vi "校准任务设置.vi"(9 "精度":dbl=4.0, 10 "模型":enum32{"线性", "多项式"}(ring), 11 "用户事件":refnum<user-event>) -> ()   [LabVIEW 2016, in "斯坦道氨氮.lvlib"]
panel:
  in  "校准任务存档":T1[](array[typedef])
  out "字符串":string
  out "校准运行状态":bool
  in  "校准任务":T1[](array[typedef])
  in  "停止":bool
  in  "设置":bool
  in  "执行":bool
  in  "删除":bool
  in  "清空":bool
  in  "任务列表":i32(listbox)
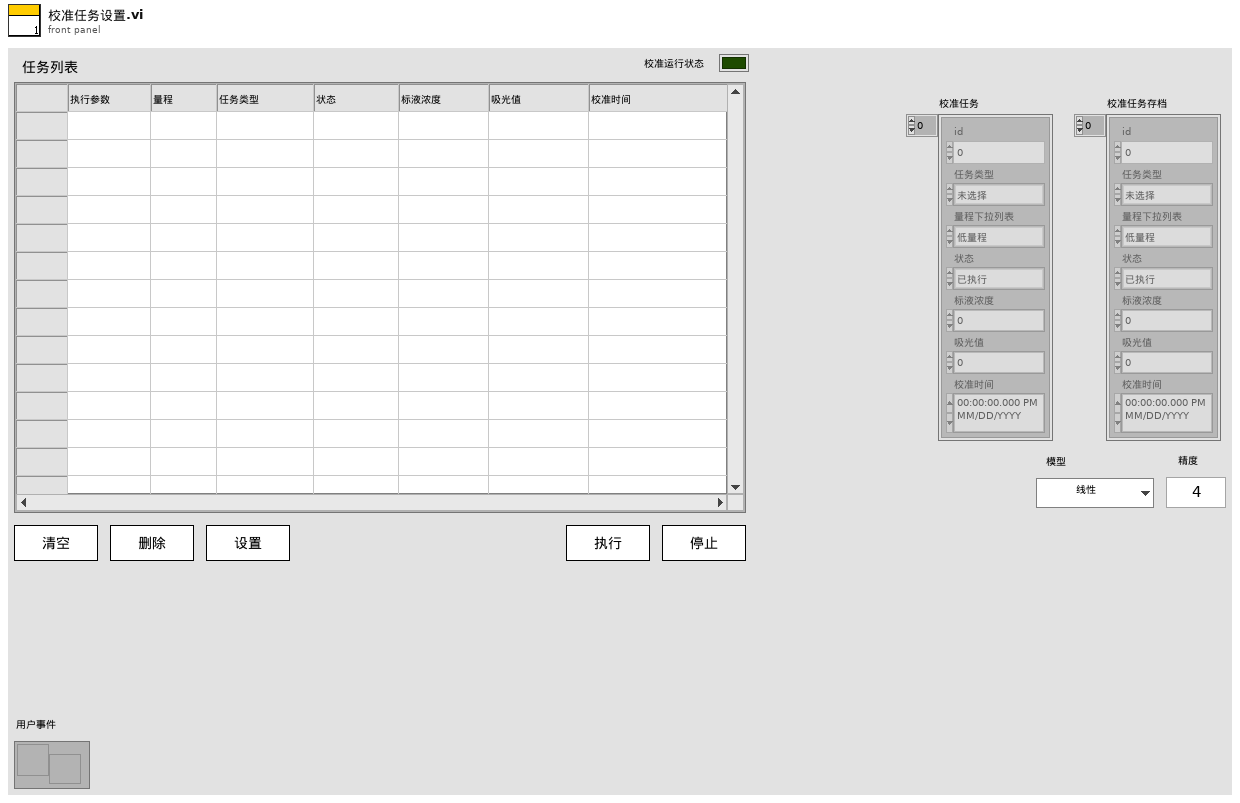
[diagram p1: front panel]
types:
  T1 = typedef "斯坦道氨氮.lvlib/校准任务.ctl" = cluster{"id":u16, "任务类型":enum16{"未选择", "空白校准", "标样校准", "标样核查", "零点核查", "跨度核查"}, "量程下拉列表":enum16{"低量程", "高量程"}, "状态":enum16{"已执行", "待执行", "执行中", "停止"}, "标液浓度":dbl, "吸光值":dbl, "校准时间":timestamp}
  T2 = cluster{"校准类型":string, "校准数据":cluster{"时间":timestamp, "标液值":dbl, "检测值":dbl, "吸光值":dbl}}
  T3 = enum8{"Enabled", "Disabled", "Disabled and Grayed Out"}
  T4 = typedef "LVPoint32TypeDef.ctl" = cluster{"Horizontal":i32, "Vertical":i32}
  T5 = typedef "LVRowAndColumnTypeDef.ctl" = cluster{"Row":i32, "Column":i32}
  T6 = enum16{"未选择", "空白校准", "标样校准", "标样核查", "零点核查", "跨度核查"}
  T7 = cluster{"id":u16, "任务类型":enum16{"未选择", "空白校准", "标样校准", "标样核查", "零点核查", "跨度核查"}, "量程下拉列表":enum16{"低量程", "高量程"}, "状态":enum16{"已执行", "待执行", "执行中", "停止"}, "标液浓度":dbl, "吸光值":dbl, "校准时间":timestamp}
  T8 = enum32{"Bad", "Idle", "Run top level", "Running"}
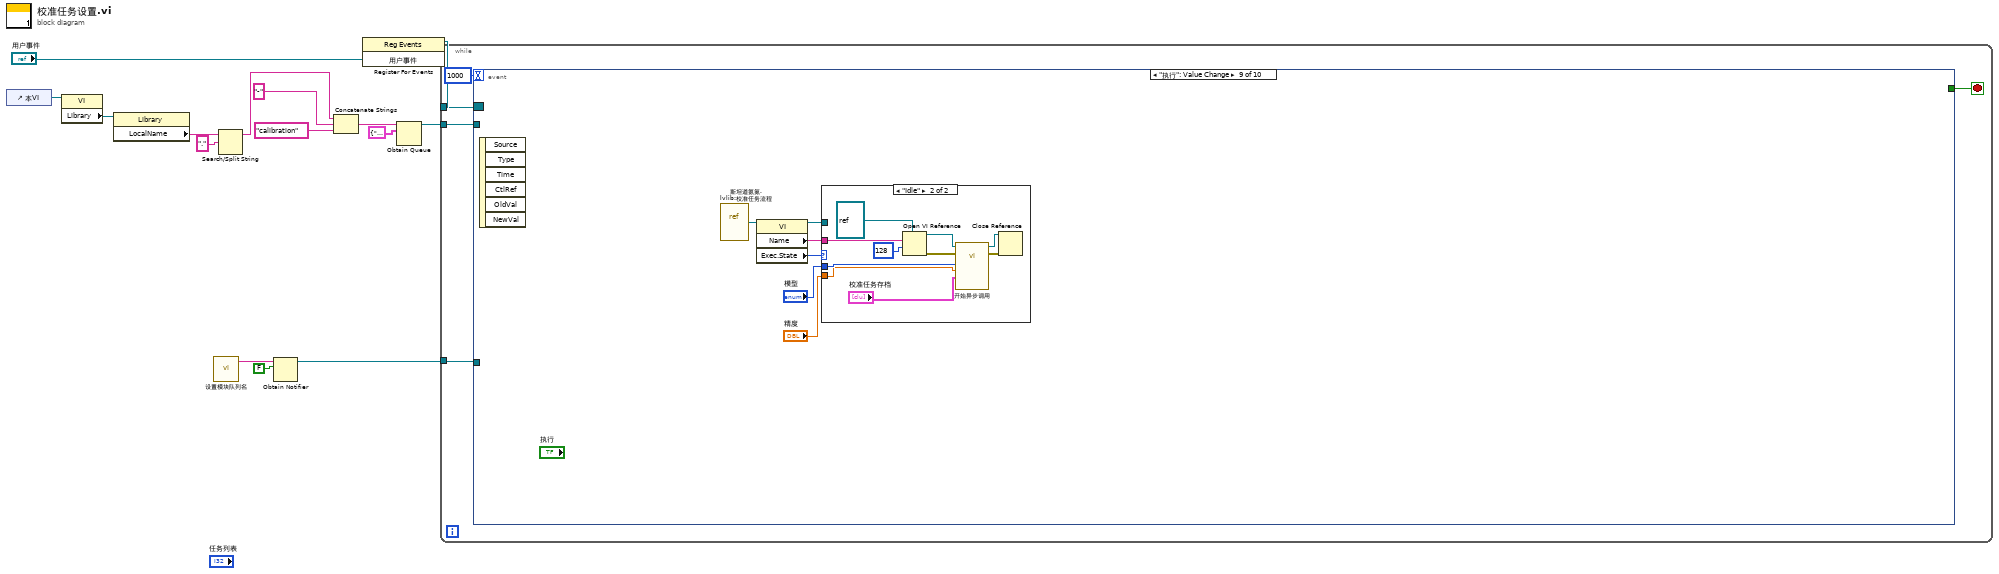
[diagram p0: block diagram]
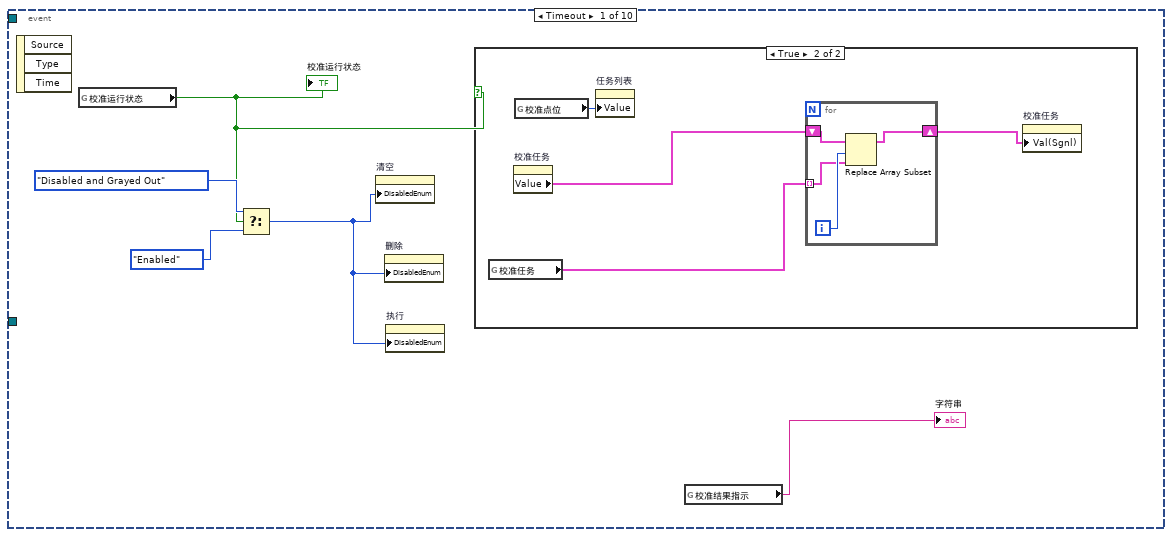
[diagram p2: hidden frame]
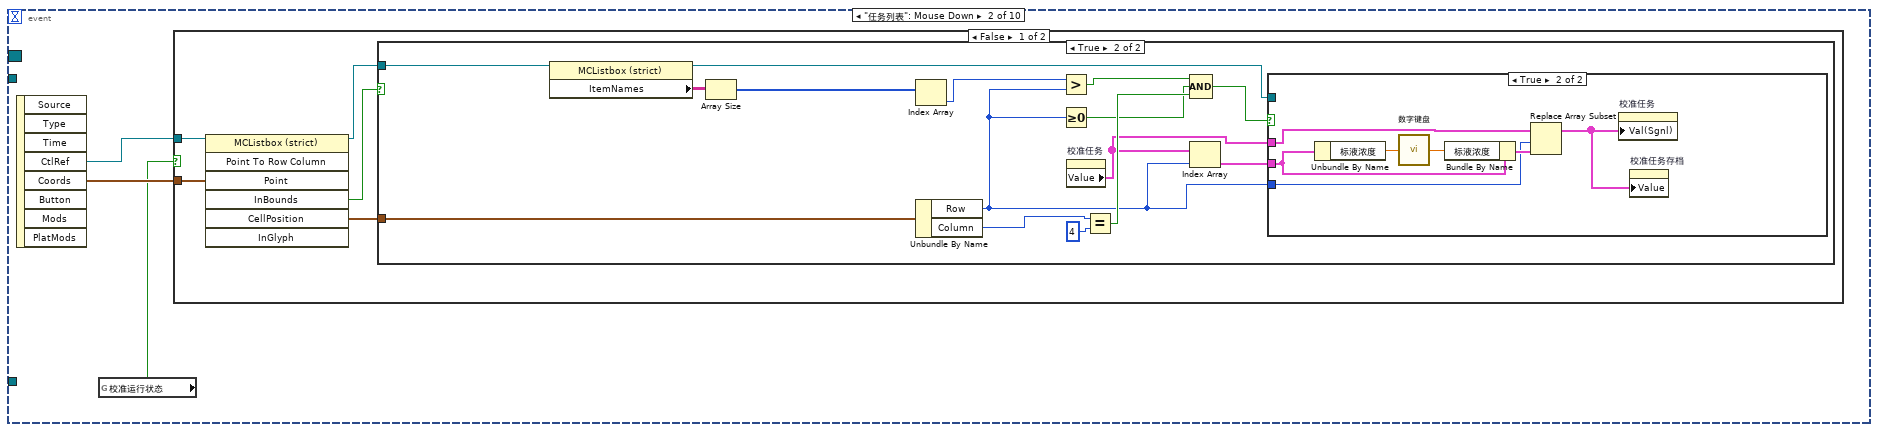
[diagram p4: hidden frame]
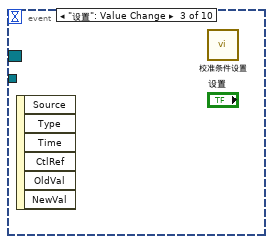
[diagram p8: hidden frame]
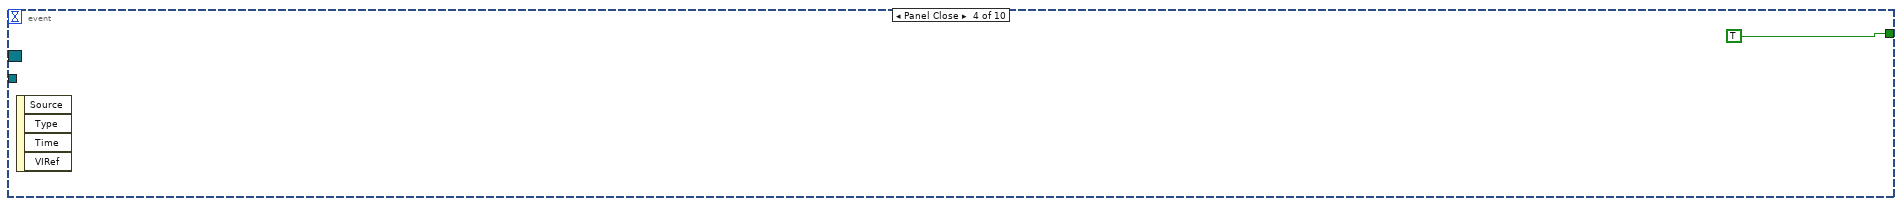
[diagram p9: hidden frame]
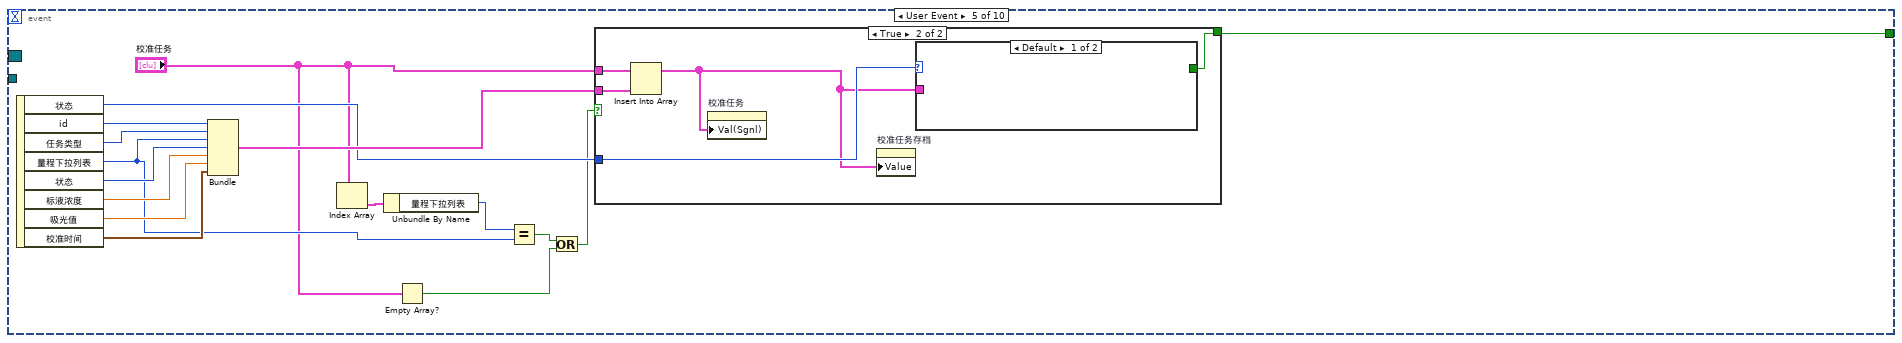
[diagram p10: hidden frame]
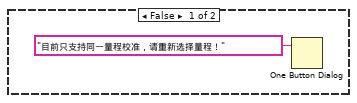
[diagram p11: hidden frame]
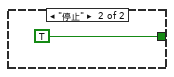
[diagram p12: hidden frame]
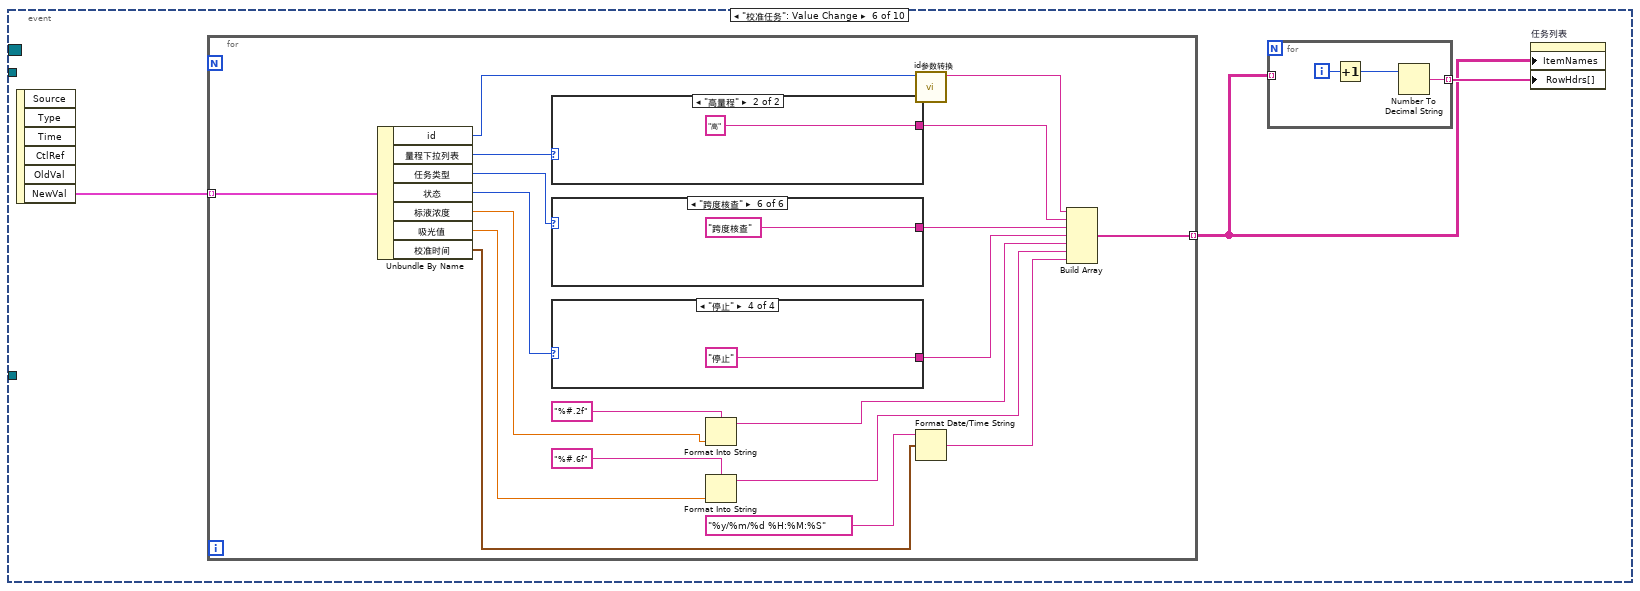
[diagram p13: hidden frame]
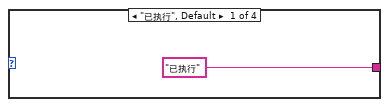
[diagram p14: hidden frame]
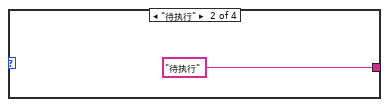
[diagram p15: hidden frame]
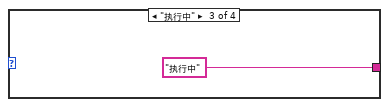
[diagram p16: hidden frame]
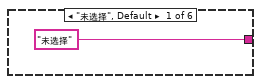
[diagram p17: hidden frame]
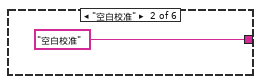
[diagram p18: hidden frame]
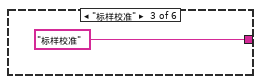
[diagram p19: hidden frame]
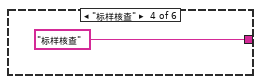
[diagram p20: hidden frame]
diagram:
  n1 = control-ref of="本VI"() -> (w14:refnum<vi>)
  n2 = property class="VI"(reference=w14) -> ("Library"=w15:refnum<vi>)  [unwired: 1 in, 2 out]
  n3 = property class="Library"(reference=w15) -> ("LocalName"=w13:string)  [unwired: 1 in, 2 out]
  n4 = call "设置模块队列名.vi"() -> ("Msg"=w2:string)  [unwired: 5 in]
  n5 = Search/Split String(string=w13, search string/char (-)="." ("搜索字符串/字符(-)")) -> (substring before match=w11:string)  [unwired: 1 in, 2 out]
  n6 = Obtain Notifier(name (unnamed)=w2, notification data type=FALSE) -> (notifier out=w1:refnum<notifier>)  [unwired: 2 in, 2 out]
  n7 = Concatenate Strings(w11, "-" ("字符串"), "calibration" ("名称或相对路径")) -> (w8:string)
  n8 = register-events("用户事件") -> (reference out=w5:refnum<event-registration>)  [unwired: 2 in, 1 out]
  n9 = Obtain Queue(name (unnamed)=w8, element data type=T2 {"校准类型"="", "校准数据"={"时间"=timestamp(0 s since 1904-01-01), "标液值"=0.0, "检测值"=0.0, "吸光值"=0.0}}) -> (queue out=w6:refnum<queue>)  [unwired: 3 in, 2 out]
  n10 = while {
    tunnel: w6 -> [w19]
    tunnel: w5 -> [w18]
    tunnel: w1 -> [w17]
    stop <- w20 stop-if-true
    n11 = event shown="[8] \"执行\": Value Change" {
      selector: w18 -> [_ _ _ _ _ _ _ _ _ _]
      dyn-events: _ -> [_ _ _ _ _ _ _ _ _ _]
      timeout: 1000 -> [_ _ _ _ _ _ _ _ _ _]
      tunnel: [_ _ _ TRUE w80 _ _ _ _ _] -> w20
      tunnel: w19 -> [_ _ _ _ _ _ _ _ _ _]
      tunnel: w17 -> [_ _ _ _ _ _ _ _ _ w146]
      event Timeout {
        n12 = event-data() -> ()  [unwired: 1 in, 3 out]
        n13 = global read "VAR总磷总氮全局变量.vi" "校准运行状态"() -> (w22:bool)
        "校准运行状态" <- w22
        n14 = Select(t=T3."Disabled and Grayed Out" ("禁用"), s=w22, f=T3."Enabled" ("禁用")) -> (s? t:f=w24:T3)
        n15 = property on="清空" class="Bool"("DisabledEnum"=w24) -> ()  [unwired: 2 in, 2 out]
        n16 = property on="删除" class="Bool"("DisabledEnum"=w24) -> ()  [unwired: 2 in, 2 out]
        n17 = property on="执行" class="Bool"("DisabledEnum"=w24) -> ()  [unwired: 2 in, 2 out]
        n18 = case shown="True" w22 {
          frame False {
          }
          frame True {
            n19 = global read "VAR总磷总氮全局变量.vi" "校准任务"() -> (w27:T1[])
            n20 = property on="校准任务" class="Arr (strict)"() -> ("Value"=w28:T1[])  [unwired: 2 in, 2 out]
            n21 = global read "VAR总磷总氮全局变量.vi" "校准点位"() -> (w29:u16)
            n22 = property on="任务列表" class="MCListbox (strict)"("Value"=w29) -> ()  [unwired: 2 in, 2 out]
            n23 = for {
              tunnel: w27 -> [w31] mode=indexing
              shift-right: [w30] -> w26
              shift-left: w28 -> [w33]
              i -> [w32]
              n24 = Replace Array Subset(array=w33, new element=w31, index=w32) -> (w30:T1[])
            }
            n25 = property on="校准任务" class="Arr (strict)"("Val(Sgnl)"=w26) -> ()  [unwired: 2 in, 2 out]
          }
        }
        n26 = global read "VAR总磷总氮全局变量.vi" "校准结果指示"() -> (→"字符串":string)
      }
      event "任务列表": Mouse Down {
        n27 = event-data() -> ("CtlRef"=w36:refnum<vi>, "Coords"=w35:T4)  [unwired: 1 in, 6 out]
        n28 = global read "VAR总磷总氮全局变量.vi" "校准运行状态"() -> (w34:bool)
        n29 = case shown="False" w34 {
          tunnel: w36 -> [w41 _]
          tunnel: w35 -> [w37 _]
          frame False {
            n30 = invoke class="MCListbox (strict)" method="Point To Row Column"(reference=w41, "Point"=w37) -> (reference out=w38:refnum<vi>, "InBounds"=w40:bool, "CellPosition"=w39:T5)  [unwired: 5 in, 4 out]
            n31 = case shown="True" w40 {
              tunnel: w39 -> [_ w56]
              tunnel: w38 -> [_ w55]
              frame False {
              }
              frame True {
                n32 = property class="MCListbox (strict)"(reference=w55) -> (reference out=w54:refnum<vi>, "ItemNames"=w53:string[][])  [unwired: 1 in, 1 out]
                n33 = Array Size(array=w53) -> (size(s)=w52:i32[])
                n34 = Index Array(array=w52) -> (element=w51:i32)  [unwired: 1 in]
                n35 = Unbundle By Name(w56) -> ("Row"=w42:i32, "Column"=w50:i32)
                n36 = Greater?(x=w51, y=w42) -> (0:w46:bool)
                n37 = Greater Or Equal To 0?(x=w42) -> (x >= 0?=w45:bool)
                n38 = property on="校准任务" class="Arr (strict)"() -> ("Value"=w43:T1[])  [unwired: 2 in, 2 out]
                n39 = Equal?(x=w50, y=4) -> (x = y?=w48:bool)
                n40 = Compound Arithmetic op=AND ("复合运算")(w46, w45, w48) -> (w47:bool)
                n41 = Index Array(array=w43, index=w42) -> (element=w44:T1)
                n42 = case shown="True" w47 {
                  tunnel: w54 -> [_ _]
                  tunnel: w44 -> [_ w62]
                  tunnel: w43 -> [_ w60]
                  tunnel: w42 -> [_ w58]
                  frame False {
                  }
                  frame True {
                    n43 = Unbundle By Name(w62) -> ("标液浓度"=w63:dbl)
                    n44 = call "数字键盘.vi"("OldNumber"=w63) -> ("NewNumber"=w61:dbl)
                    n45 = Bundle By Name(cluster=w62, "标液浓度"=w61) -> (w59:T1)
                    n46 = Replace Array Subset(array=w60, new element=w59, index=w58) -> (w57:T1[])
                    n47 = property on="校准任务" class="Arr (strict)"("Val(Sgnl)"=w57) -> ()  [unwired: 2 in, 2 out]
                    n48 = property on="校准任务存档" class="Arr (strict)"("Value"=w57) -> ()  [unwired: 2 in, 2 out]
                  }
                }
              }
            }
          }
          frame True {
          }
        }
      }
      event "设置": Value Change {
        n49 = event-data() -> ()  [unwired: 1 in, 6 out]
        n50 = call "校准条件设置.vi"() -> ()  [unwired: 12 in]
      }
      event Panel Close {
        n51 = event-data() -> ()  [unwired: 1 in, 4 out]
      }
      event User Event {
        n52 = event-data() -> ("状态"=w72:enum16{"已执行", "待执行", "执行中", "停止"}, "id"=w79:u16, "任务类型"=w77:T6, "量程下拉列表"=w69:enum16{"低量程", "高量程"}, "状态"=w76:enum16{"已执行", "待执行", "执行中", "停止"}, "标液浓度"=w75:dbl, "吸光值"=w74:dbl, "校准时间"=w73:timestamp)  [unwired: 1 in]
        n53 = Bundle("id"=w79, "任务类型"=w77, "量程下拉列表"=w69, "状态"=w76, "标液浓度"=w75, "吸光值"=w74, "校准时间"=w73) -> (w78:T7)  [unwired: 1 in]
        n54 = Index Array(array="校准任务") -> (element=w71:T1)  [unwired: 1 in]
        n55 = Unbundle By Name(w71) -> ("量程下拉列表"=w70:enum16{"低量程", "高量程"})
        n56 = Empty Array?(array="校准任务") -> (empty?=w65:bool)
        n57 = Equal?(x=w70, y=w69) -> (x = y?=w67:bool)
        n58 = Or(x=w67, y=w65) -> (x .or. y?=w66:bool)
        n59 = case shown="True" w66 {
          tunnel: [_ w86] -> w80
          tunnel: w78 -> [_ w85]
          tunnel: w72 -> [_ w84]
          tunnel: "校准任务" -> [_ w83]
          frame False {
            n60 = One Button Dialog(message="目前只支持同一量程校准，请重新选择量程！" ("消息")) -> ()  [unwired: 1 in, 1 out]
          }
          frame True {
            n61 = Insert Into Array(array=w83, new element=w85) -> (w82:T1[])  [unwired: 1 in]
            n62 = property on="校准任务" class="Arr (strict)"("Val(Sgnl)"=w82) -> ()  [unwired: 2 in, 2 out]
            n63 = property on="校准任务存档" class="Arr (strict)"("Value"=w82) -> ()  [unwired: 2 in, 2 out]
            n64 = case shown="Default" w84 {
              tunnel: [_ TRUE] -> w86
              tunnel: w82 -> [_ _]
              frame Default {
              }
              frame "停止" {
              }
            }
          }
        }
      }
      event "校准任务": Value Change {
        n65 = event-data() -> ("NewVal"=w88:T1[])  [unwired: 1 in, 5 out]
        n66 = for {
          tunnel: w88 -> [w109] mode=indexing
          tunnel: [w91] -> w89 mode=indexing
          n67 = Unbundle By Name(w109) -> ("id"=w108:u16, "量程下拉列表"=w107:enum16{"低量程", "高量程"}, "任务类型"=w106:T6, "状态"=w105:enum16{"已执行", "待执行", "执行中", "停止"}, "标液浓度"=w103:dbl, "吸光值"=w101:dbl, "校准时间"=w99:timestamp)
          n68 = case shown="\"高量程\"" w107 {
            tunnel: ["低" "高"] -> w97
            frame "低量程", Default {
            }
            frame "高量程" {
            }
          }
          n69 = case shown="\"跨度核查\"" w106 {
            tunnel: ["未选择" "空白校准" "标样校准" "标样核查" "零点核查" "跨度核查"] -> w96
            frame "未选择", Default {
            }
            frame "空白校准" {
            }
            frame "标样校准" {
            }
            frame "标样核查" {
            }
            frame "零点核查" {
            }
            frame "跨度核查" {
            }
          }
          n70 = case shown="\"停止\"" w105 {
            tunnel: ["已执行" "待执行" "执行中" "停止"] -> w95
            frame "已执行", Default {
            }
            frame "待执行" {
            }
            frame "执行中" {
            }
            frame "停止" {
            }
          }
          n71 = Format Into String(format string="%#.2f" ("格式字符串"), w103) -> (resulting string=w94:string)  [unwired: 2 in, 1 out]
          n72 = Format Into String(format string="%#.6f" ("格式字符串"), w101) -> (resulting string=w93:string)  [unwired: 2 in, 1 out]
          n73 = call "id参数转换.vi"("id"=w108) -> ("table输出"=w98:string)  [unwired: 9 in, 1 out]
          n74 = Format Date/Time String(time format string (%c)="%y/%m/%d %H:%M:%S" ("时间格式字符串(%c)"), seconds (now)=w99) -> (date/time string=w92:string)  [unwired: 1 in]
          n75 = Build Array(w98, w97, w96, w95, w94, w93, w92) -> (w91:string[])
        }
        n76 = for {
          tunnel: [w122] -> w90 mode=indexing
          tunnel: w89 -> [_] mode=indexing
          i -> [w124]
          n77 = Increment(x=w124) -> (x+1=w123:i32)
          n78 = Number To Decimal String(number=w123) -> (decimal integer string=w122:string)  [unwired: 1 in]
        }
        n79 = property on="任务列表" class="MCListbox (strict)"("ItemNames"=w89, "RowHdrs[]"=w90) -> ()  [unwired: 2 in, 2 out]
      }
      event "清空": Value Change {
        n80 = event-data() -> ()  [unwired: 1 in, 6 out]
        n81 = property on="校准任务" class="Arr (strict)"("Val(Sgnl)"=T1[] [] ("数组")) -> ()  [unwired: 2 in, 2 out]
      }
      event "删除": Value Change {
        n82 = event-data() -> ()  [unwired: 1 in, 6 out]
        n83 = property on="校准任务" class="Arr (strict)"() -> ("Value"=w128:T1[])  [unwired: 2 in, 2 out]
        n84 = property on="任务列表" class="MCListbox (strict)"() -> ("Value"=w126:i32)  [unwired: 2 in, 2 out]
        n85 = Delete From Array(array=w128, index=w126) -> (array with subset deleted=w127:T1[])  [unwired: 1 in, 1 out]
        n86 = property on="校准任务" class="Arr (strict)"("Val(Sgnl)"=w127) -> ()  [unwired: 2 in, 2 out]
      }
      event "执行": Value Change {
        n87 = event-data() -> ()  [unwired: 1 in, 6 out]
        n88 = vi-ref "斯坦道氨氮.lvlib:校准任务流程.vi"() -> (w131:refnum<vi>)
        n89 = property class="VI"(reference=w131) -> (reference out=w134:refnum<vi>, "Name"=w132:string, "Exec.State"=w133:T8)  [unwired: 1 in, 1 out]
        n90 = case shown="\"Idle\"" w133 {
          tunnel: w132 -> [_ w144]
          tunnel: w134 -> [_ _]
          tunnel: "模型" -> [_ w137]
          tunnel: "精度" -> [_ w136]
          frame "Bad", Default {
          }
          frame "Idle" {
            n91 = Open VI Reference(type specifier VI Refnum (for type only)=refnum<vi> refnum, vi path=w144, options=128 ("选项")) -> (vi reference=w142:refnum<vi>, error out=w140:errorcluster)  [unwired: 3 in]
            n92 = call-by-ref "开始异步调用"(reference=w142, error in=w140, "校准任务"="校准任务存档", "精度"=w136, "模型"=w137) -> (reference out=w141:refnum<vi>, error out=w139:errorcluster)  [unwired: 9 in]
            n93 = Close Reference(reference=w141, error in (no error)=w139) -> ()  [unwired: 1 out]
          }
        }
      }
      event "停止": Value Change {
        n94 = event-data() -> ()  [unwired: 1 in, 6 out]
        n95 = Send Notification(notification=TRUE ("通知"), notifier=w146) -> ()  [unwired: 1 in, 2 out]
      }
    }
  }
